vi "Untitled 1.vi"() -> ()   [LabVIEW 2017]
panel:
  out "AVI Path":path=path "u:/media/sdc1/data_log"
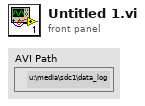
[diagram p1: front panel]
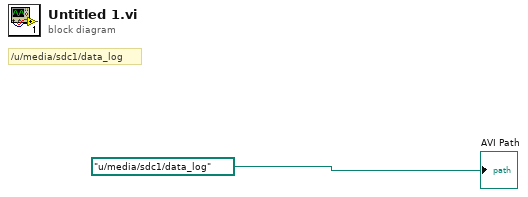
[diagram p0: block diagram]
diagram:
  # "/u/media/sdc1/data_log"
  "AVI Path" <- path "u:/media/sdc1/data_log" ("AVI Path")
